vi "ex5.vi"() -> ()   [LabVIEW 2019]
panel:
  out "cluster1 4":cluster{"1":bool, "2":bool, "3":bool}
  out "cluster1 3":cluster{"1":bool, "2":bool, "3":bool}
  out "cluster1 2":cluster{"1":bool, "2":bool, "3":bool}
  out "cluster1":cluster{"1":bool, "2":bool, "3":bool}
  out "1":bool
  out "3.2":bool
  out "3.1":bool
  out "3.3":bool
  out "1.3":bool
  out "1.2":bool
  out "1.1":bool
  out "2":bool
  out "3":bool
  out "2.2":bool
  out "2.3":bool
  out "2.1":bool
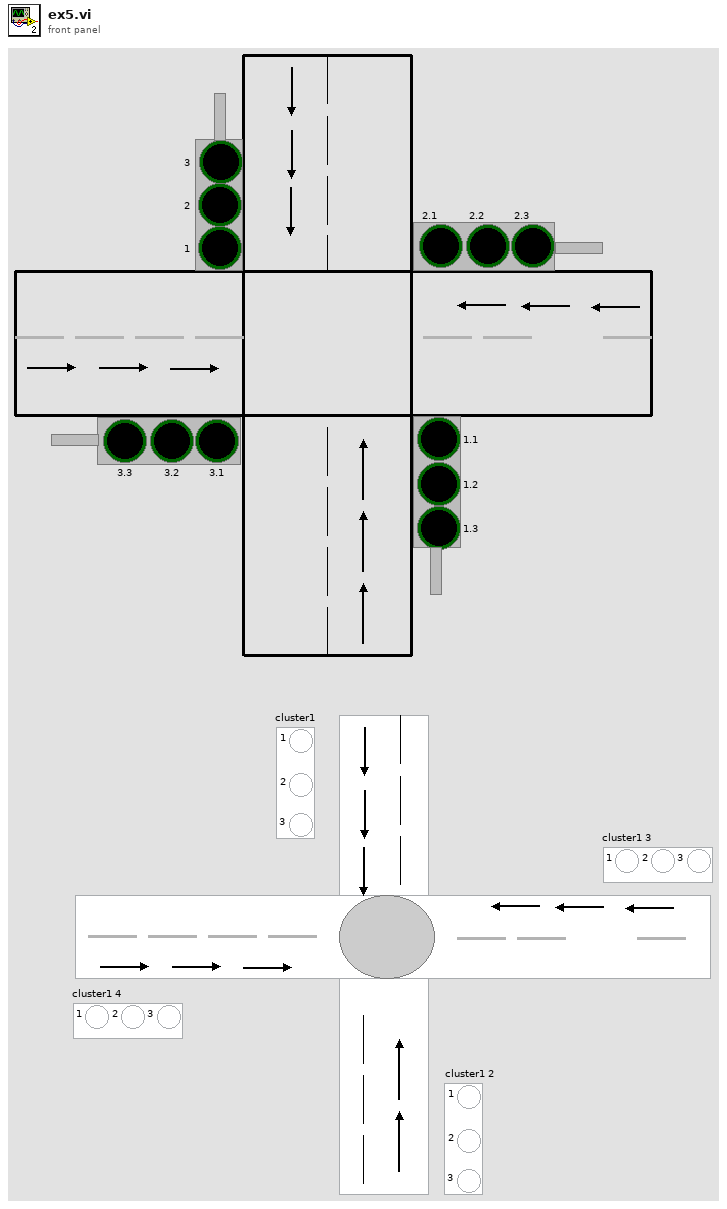
[diagram p1: front panel]
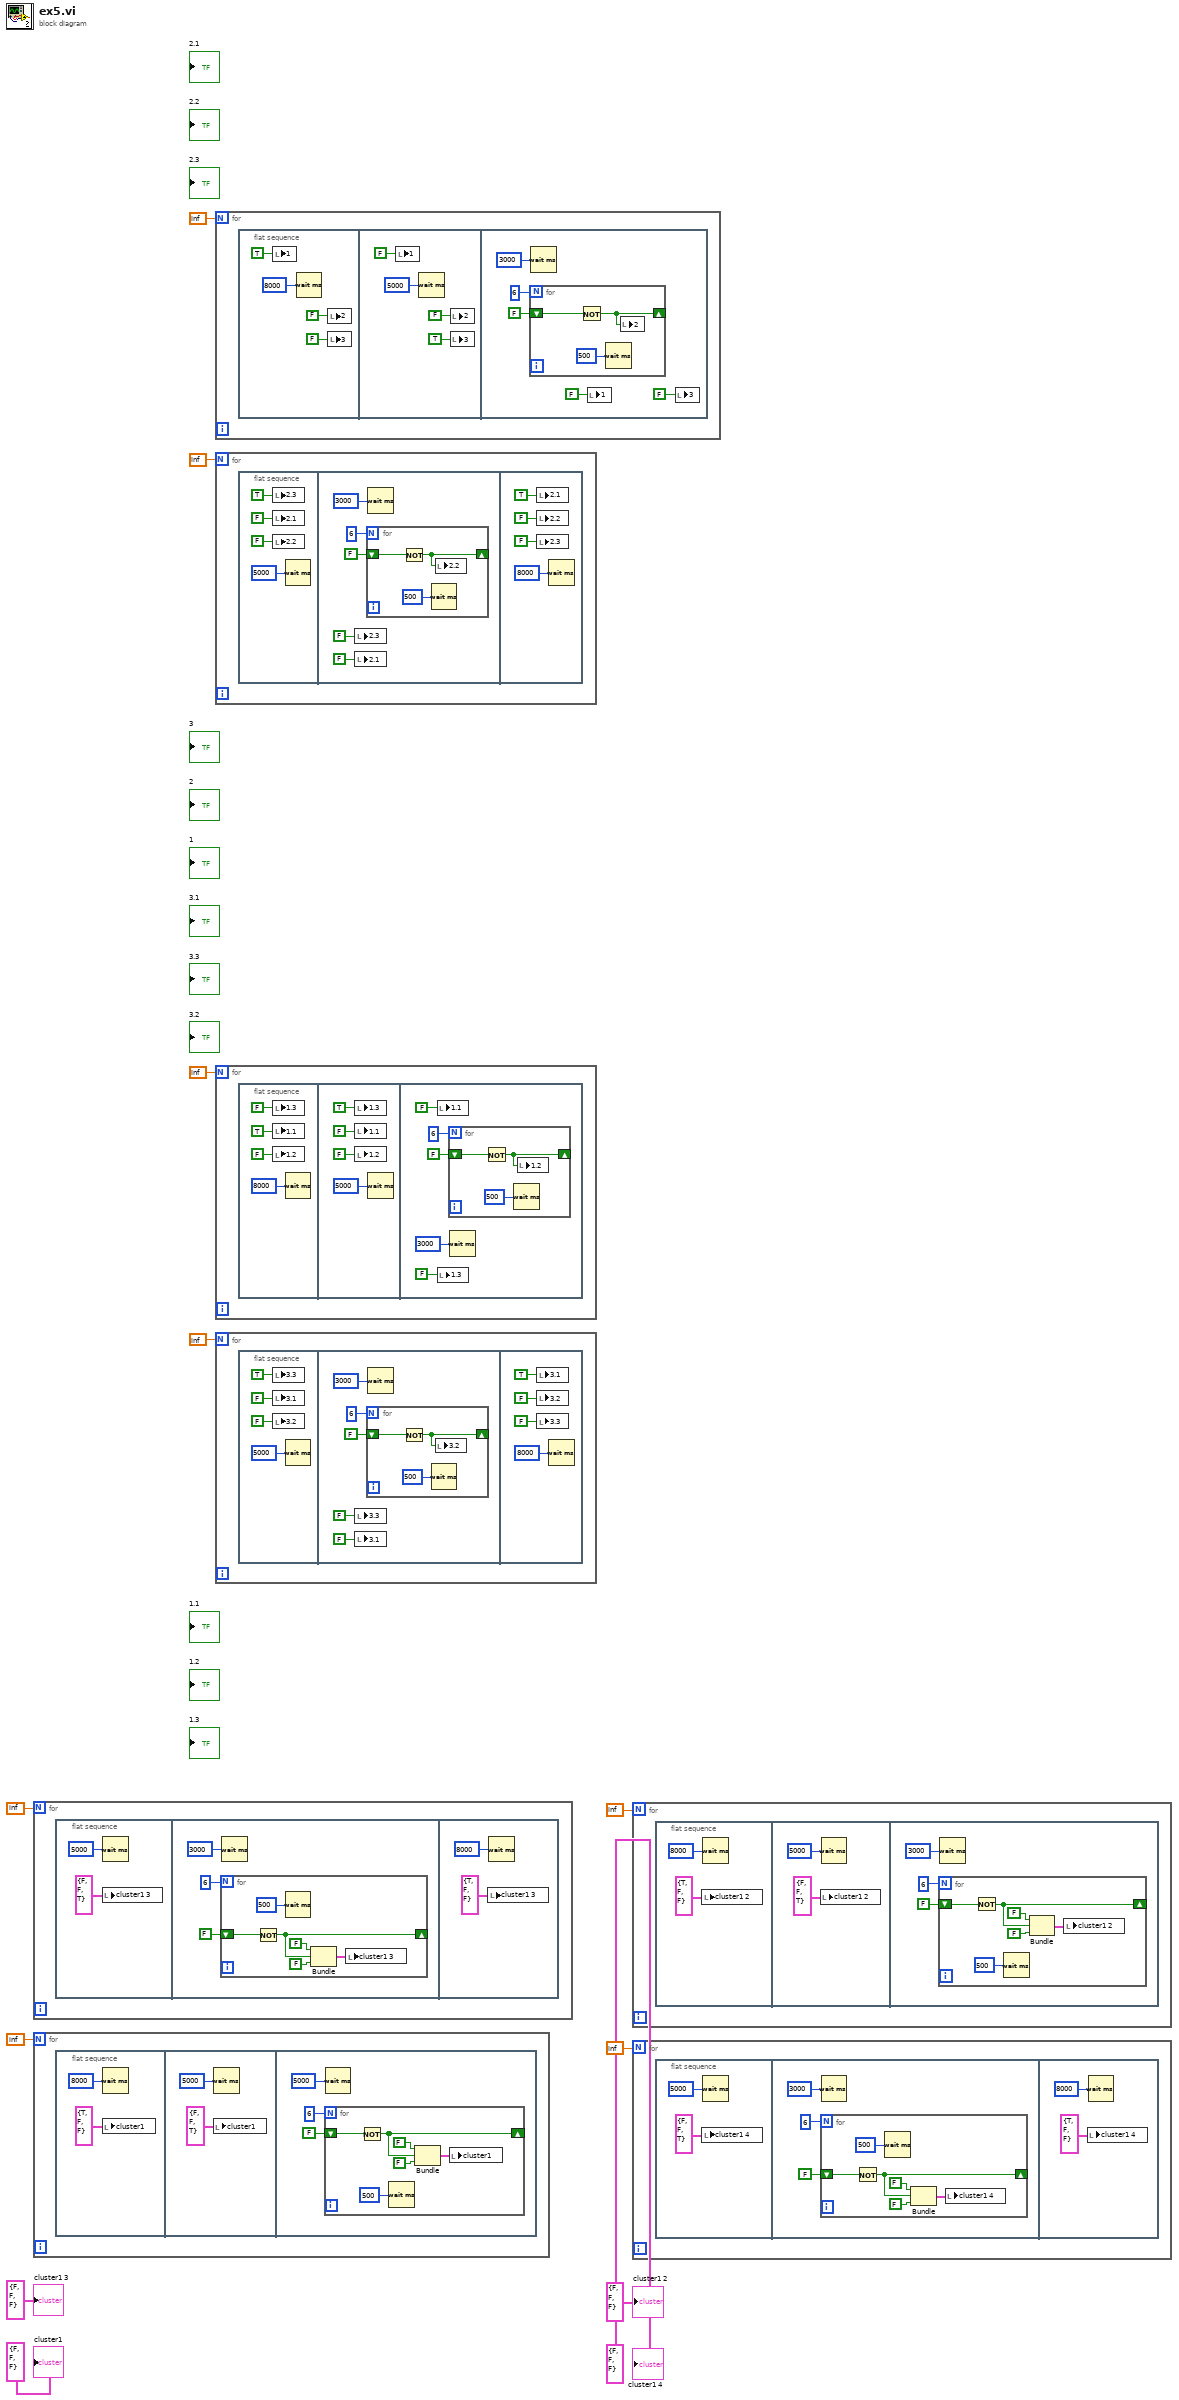
[diagram p0: block diagram]
diagram:
  n1 = for {
    N: inf -> [_]
    n2 = flat-sequence {
      frame #0 {
        n3 = local write "cluster1 3"(cluster{"1":bool, "2":bool, "3":bool} {"1"=FALSE, "2"=FALSE, "3"=TRUE} ("cluster1")) -> ()
        n4 = Wait (ms)(milliseconds to wait=5000) -> ()  [unwired: 1 out]
      }
      frame #1 {
        n5 = for {
          N: 6 -> [_]
          shift-right: [w21] -> _
          shift-left: FALSE -> [w23]
          n6 = Not(x=w23) -> (.not. x?=w21:bool)
          n7 = Wait (ms)(milliseconds to wait=500) -> ()  [unwired: 1 out]
          n8 = Bundle(FALSE, w21, FALSE) -> (w20:cluster{bool, bool, bool})  [unwired: 1 in]
          n9 = local write "cluster1 3"(w20) -> ()
        }
        n10 = Wait (ms)(milliseconds to wait=3000) -> ()  [unwired: 1 out]
      }
      frame #2 {
        n11 = local write "cluster1 3"(cluster{"1":bool, "2":bool, "3":bool} {"1"=TRUE, "2"=FALSE, "3"=FALSE} ("cluster1")) -> ()
        n12 = Wait (ms)(milliseconds to wait=8000) -> ()  [unwired: 1 out]
      }
    }
  }
  n13 = for {
    N: inf -> [_]
    n14 = flat-sequence {
      frame #0 {
        n15 = local write "cluster1"(cluster{"1":bool, "2":bool, "3":bool} {"1"=TRUE, "2"=FALSE, "3"=FALSE} ("cluster1")) -> ()
        n16 = Wait (ms)(milliseconds to wait=8000) -> ()  [unwired: 1 out]
      }
      frame #1 {
        n17 = local write "cluster1"(cluster{"1":bool, "2":bool, "3":bool} {"1"=FALSE, "2"=FALSE, "3"=TRUE} ("cluster1")) -> ()
        n18 = Wait (ms)(milliseconds to wait=5000) -> ()  [unwired: 1 out]
      }
      frame #2 {
        n19 = for {
          N: 6 -> [_]
          shift-right: [w36] -> _
          shift-left: FALSE -> [w38]
          n20 = Not(x=w38) -> (.not. x?=w36:bool)
          n21 = Wait (ms)(milliseconds to wait=500) -> ()  [unwired: 1 out]
          n22 = Bundle(FALSE, w36, FALSE) -> (w35:cluster{bool, bool, bool})  [unwired: 1 in]
          n23 = local write "cluster1"(w35) -> ()
        }
        n24 = Wait (ms)(milliseconds to wait=5000) -> ()  [unwired: 1 out]
      }
    }
  }
  n25 = for {
    N: inf -> [_]
    n26 = flat-sequence {
      frame #0 {
        n27 = local write "1"(TRUE) -> ()
        n28 = Wait (ms)(milliseconds to wait=8000) -> ()  [unwired: 1 out]
        n29 = local write "2"(FALSE) -> ()
        n30 = local write "3"(FALSE) -> ()
      }
      frame #1 {
        n31 = local write "1"(FALSE) -> ()
        n32 = Wait (ms)(milliseconds to wait=5000) -> ()  [unwired: 1 out]
        n33 = local write "2"(FALSE) -> ()
        n34 = local write "3"(TRUE) -> ()
      }
      frame #2 {
        n35 = for {
          N: 6 -> [_]
          shift-right: [w53] -> _
          shift-left: FALSE -> [w54]
          n36 = Not(x=w54) -> (.not. x?=w53:bool)
          n37 = Wait (ms)(milliseconds to wait=500) -> ()  [unwired: 1 out]
          n38 = local write "2"(w53) -> ()
        }
        n39 = Wait (ms)(milliseconds to wait=3000) -> ()  [unwired: 1 out]
        n40 = local write "1"(FALSE) -> ()
        n41 = local write "3"(FALSE) -> ()
      }
    }
  }
  n42 = for {
    N: inf -> [_]
    n43 = flat-sequence {
      frame #0 {
        n44 = local write "2.3"(TRUE) -> ()
        n45 = local write "2.1"(FALSE) -> ()
        n46 = local write "2.2"(FALSE) -> ()
        n47 = Wait (ms)(milliseconds to wait=5000) -> ()  [unwired: 1 out]
      }
      frame #1 {
        n48 = local write "2.3"(FALSE) -> ()
        n49 = local write "2.1"(FALSE) -> ()
        n50 = for {
          N: 6 -> [_]
          shift-right: [w65] -> _
          shift-left: FALSE -> [w66]
          n51 = Not(x=w66) -> (.not. x?=w65:bool)
          n52 = Wait (ms)(milliseconds to wait=500) -> ()  [unwired: 1 out]
          n53 = local write "2.2"(w65) -> ()
        }
        n54 = Wait (ms)(milliseconds to wait=3000) -> ()  [unwired: 1 out]
      }
      frame #2 {
        n55 = local write "2.1"(TRUE) -> ()
        n56 = local write "2.2"(FALSE) -> ()
        n57 = local write "2.3"(FALSE) -> ()
        n58 = Wait (ms)(milliseconds to wait=8000) -> ()  [unwired: 1 out]
      }
    }
  }
  n59 = for {
    N: inf -> [_]
    n60 = flat-sequence {
      frame #0 {
        n61 = local write "1.3"(FALSE) -> ()
        n62 = local write "1.1"(TRUE) -> ()
        n63 = local write "1.2"(FALSE) -> ()
        n64 = Wait (ms)(milliseconds to wait=8000) -> ()  [unwired: 1 out]
      }
      frame #1 {
        n65 = local write "1.3"(TRUE) -> ()
        n66 = local write "1.1"(FALSE) -> ()
        n67 = local write "1.2"(FALSE) -> ()
        n68 = Wait (ms)(milliseconds to wait=5000) -> ()  [unwired: 1 out]
      }
      frame #2 {
        n69 = local write "1.1"(FALSE) -> ()
        n70 = local write "1.3"(FALSE) -> ()
        n71 = for {
          N: 6 -> [_]
          shift-right: [w85] -> _
          shift-left: FALSE -> [w86]
          n72 = Not(x=w86) -> (.not. x?=w85:bool)
          n73 = Wait (ms)(milliseconds to wait=500) -> ()  [unwired: 1 out]
          n74 = local write "1.2"(w85) -> ()
        }
        n75 = Wait (ms)(milliseconds to wait=3000) -> ()  [unwired: 1 out]
      }
    }
  }
  n76 = for {
    N: inf -> [_]
    n77 = flat-sequence {
      frame #0 {
        n78 = local write "3.3"(TRUE) -> ()
        n79 = local write "3.1"(FALSE) -> ()
        n80 = local write "3.2"(FALSE) -> ()
        n81 = Wait (ms)(milliseconds to wait=5000) -> ()  [unwired: 1 out]
      }
      frame #1 {
        n82 = local write "3.3"(FALSE) -> ()
        n83 = local write "3.1"(FALSE) -> ()
        n84 = for {
          N: 6 -> [_]
          shift-right: [w97] -> _
          shift-left: FALSE -> [w98]
          n85 = Not(x=w98) -> (.not. x?=w97:bool)
          n86 = Wait (ms)(milliseconds to wait=500) -> ()  [unwired: 1 out]
          n87 = local write "3.2"(w97) -> ()
        }
        n88 = Wait (ms)(milliseconds to wait=3000) -> ()  [unwired: 1 out]
      }
      frame #2 {
        n89 = local write "3.1"(TRUE) -> ()
        n90 = local write "3.2"(FALSE) -> ()
        n91 = local write "3.3"(FALSE) -> ()
        n92 = Wait (ms)(milliseconds to wait=8000) -> ()  [unwired: 1 out]
      }
    }
  }
  n93 = for {
    N: inf -> [_]
    n94 = flat-sequence {
      frame #0 {
        n95 = local write "cluster1 2"(cluster{"1":bool, "2":bool, "3":bool} {"1"=TRUE, "2"=FALSE, "3"=FALSE} ("cluster1")) -> ()
        n96 = Wait (ms)(milliseconds to wait=8000) -> ()  [unwired: 1 out]
      }
      frame #1 {
        n97 = local write "cluster1 2"(cluster{"1":bool, "2":bool, "3":bool} {"1"=FALSE, "2"=FALSE, "3"=TRUE} ("cluster1")) -> ()
        n98 = Wait (ms)(milliseconds to wait=5000) -> ()  [unwired: 1 out]
      }
      frame #2 {
        n99 = for {
          N: 6 -> [_]
          shift-right: [w113] -> _
          shift-left: FALSE -> [w115]
          n100 = Not(x=w115) -> (.not. x?=w113:bool)
          n101 = Wait (ms)(milliseconds to wait=500) -> ()  [unwired: 1 out]
          n102 = Bundle(FALSE, w113, FALSE) -> (w112:cluster{bool, bool, bool})  [unwired: 1 in]
          n103 = local write "cluster1 2"(w112) -> ()
        }
        n104 = Wait (ms)(milliseconds to wait=3000) -> ()  [unwired: 1 out]
      }
    }
  }
  n105 = for {
    N: inf -> [_]
    n106 = flat-sequence {
      frame #0 {
        n107 = local write "cluster1 4"(cluster{"1":bool, "2":bool, "3":bool} {"1"=FALSE, "2"=FALSE, "3"=TRUE} ("cluster1")) -> ()
        n108 = Wait (ms)(milliseconds to wait=5000) -> ()  [unwired: 1 out]
      }
      frame #1 {
        n109 = for {
          N: 6 -> [_]
          shift-right: [w124] -> _
          shift-left: FALSE -> [w126]
          n110 = Not(x=w126) -> (.not. x?=w124:bool)
          n111 = Wait (ms)(milliseconds to wait=500) -> ()  [unwired: 1 out]
          n112 = Bundle(FALSE, w124, FALSE) -> (w123:cluster{bool, bool, bool})  [unwired: 1 in]
          n113 = local write "cluster1 4"(w123) -> ()
        }
        n114 = Wait (ms)(milliseconds to wait=3000) -> ()  [unwired: 1 out]
      }
      frame #2 {
        n115 = local write "cluster1 4"(cluster{"1":bool, "2":bool, "3":bool} {"1"=TRUE, "2"=FALSE, "3"=FALSE} ("cluster1")) -> ()
        n116 = Wait (ms)(milliseconds to wait=8000) -> ()  [unwired: 1 out]
      }
    }
  }
  "cluster1" <- cluster{"1":bool, "2":bool, "3":bool} {"1"=FALSE, "2"=FALSE, "3"=FALSE} ("Cluster 2")
  "cluster1 2" <- cluster{"1":bool, "2":bool, "3":bool} {"1"=FALSE, "2"=FALSE, "3"=FALSE} ("Cluster 2")
  "cluster1 3" <- cluster{"1":bool, "2":bool, "3":bool} {"1"=FALSE, "2"=FALSE, "3"=FALSE} ("Cluster 2")
  "cluster1 4" <- cluster{"1":bool, "2":bool, "3":bool} {"1"=FALSE, "2"=FALSE, "3"=FALSE} ("Cluster 2")
